vi "Step_Forward.vi"(3 "error in":errorcluster, 4 "Data in":T1, 5 "Step control reference in":refnum<vi>) -> (0 "error out":errorcluster, 1 "Data out":T1, 2 "Step control reference out":refnum<vi>)   [LabVIEW 2015]
uses:
  Type_Defs/Data.ctl
  Type_Defs/Diagnostics.ctl
  Type_Defs/Systems.ctl
  Step_Vis/Steps.lvlib
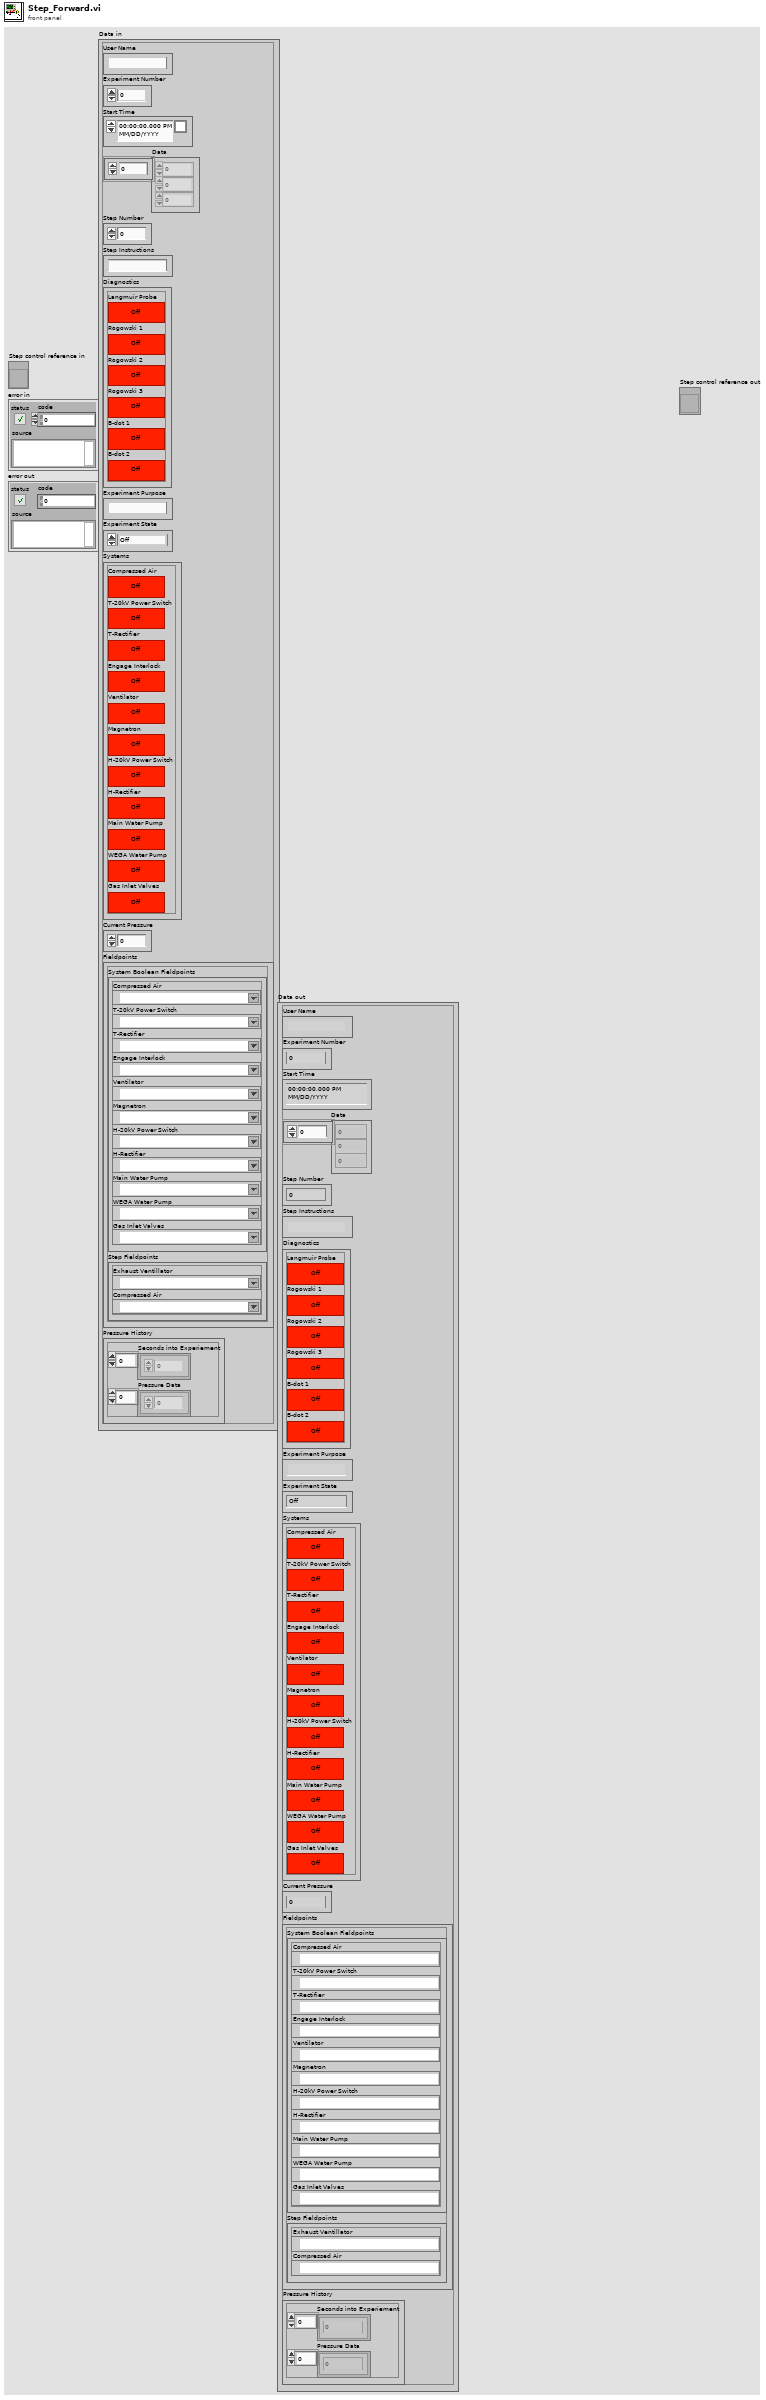
[diagram p1: front panel]
types:
  T1 = typedef "Data.ctl" = cluster{"User Name":string, "Experiment Number":i32, "Start Time":timestamp, "Data":dbl[], "Step Number":i32, "Step Instructions":string, "Diagnostics":T2, "Experiment Purpose":string, "Experiment State":enum16{"Off", "Setting Up", "Ready", "In Progress", "Shutting Down"}, "Systems":T3, "Current Pressure":dbl, "Fieldpoints":cluster{"System Boolean Fieldpoints":cluster{"Compressed Air":refnum<k21>, "T-20kV Power Switch":refnum<k21>, "T-Rectifier":refnum<k21>, "Engage Interlock":refnum<k21>, "Ventilator":refnum<k21>, "Magnetron":refnum<k21>, "H-20kV Power Switch":refnum<k21>, "H-Rectifier":refnum<k21>, "Main Water Pump":refnum<k21>, "WEGA Water Pump":refnum<k21>, "Gas Inlet Valves":refnum<k21>}, "Step Fieldpoints":cluster{"Exhaust Ventillator":refnum<k21>, "Compressed Air":refnum<k21>}}, "Pressure History":cluster{"Seconds into Experiement":i32[], "Pressure Data":dbl[]}}
  T2 = typedef "Diagnostics.ctl" = cluster{"Langmuir Probe":bool, "Rogowski 1":bool, "Rogowski 2":bool, "Rogowski 3":bool, "B-dot 1":bool, "B-dot 2":bool}
  T3 = typedef "Systems.ctl" = cluster{"Compressed Air":bool, "T-20kV Power Switch":bool, "T-Rectifier":bool, "Engage Interlock":bool, "Ventilator":bool, "Magnetron":bool, "H-20kV Power Switch":bool, "H-Rectifier":bool, "Main Water Pump":bool, "WEGA Water Pump":bool, "Gas Inlet Valves":bool}
  T4 = enum16{"Off", "Setting Up", "Ready", "In Progress", "Shutting Down"}
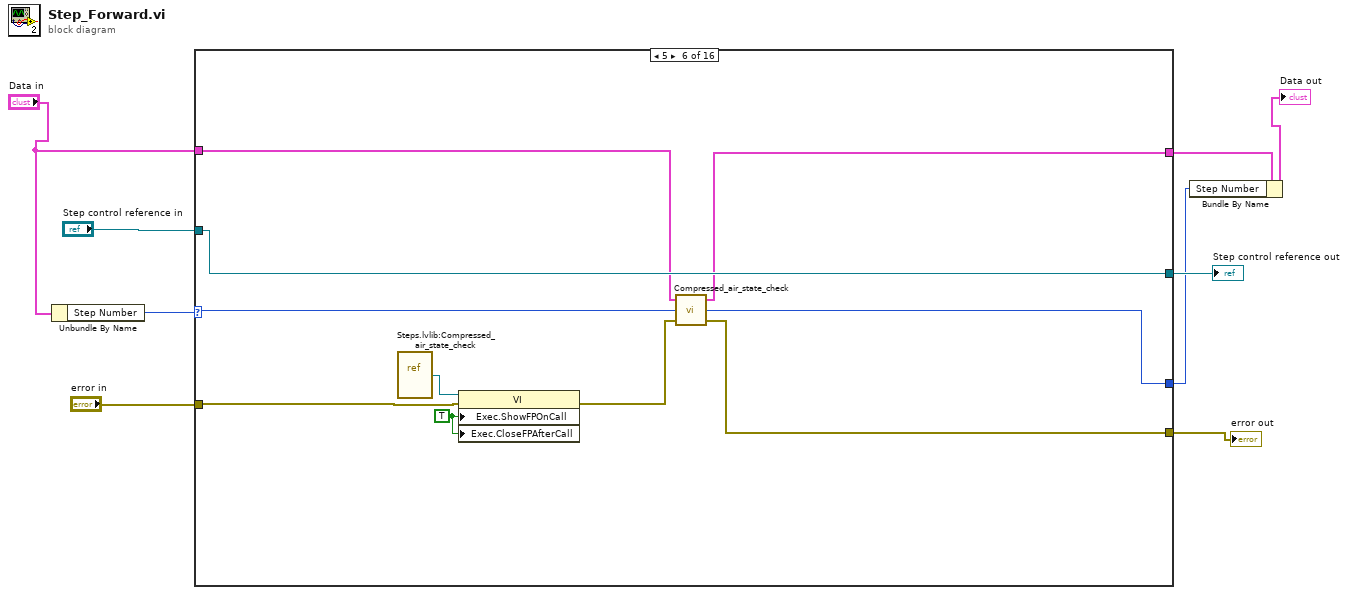
[diagram p0: block diagram]
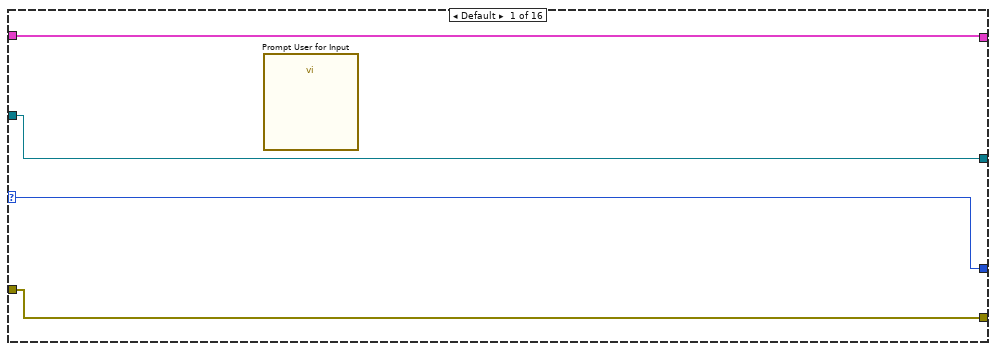
[diagram p2: hidden frame]
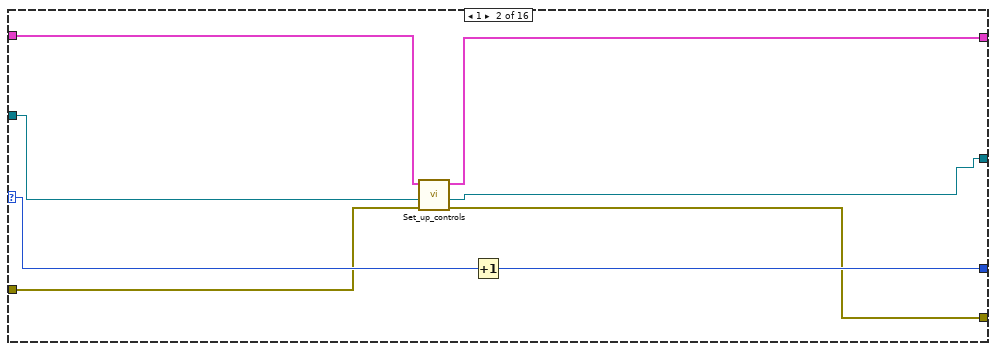
[diagram p3: hidden frame]
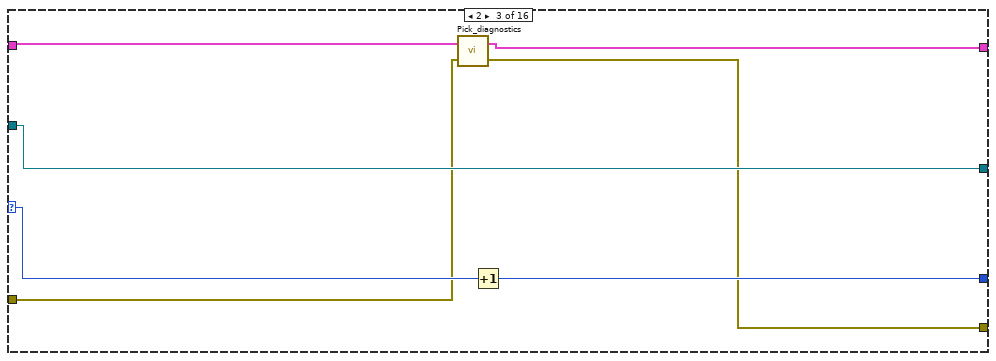
[diagram p4: hidden frame]
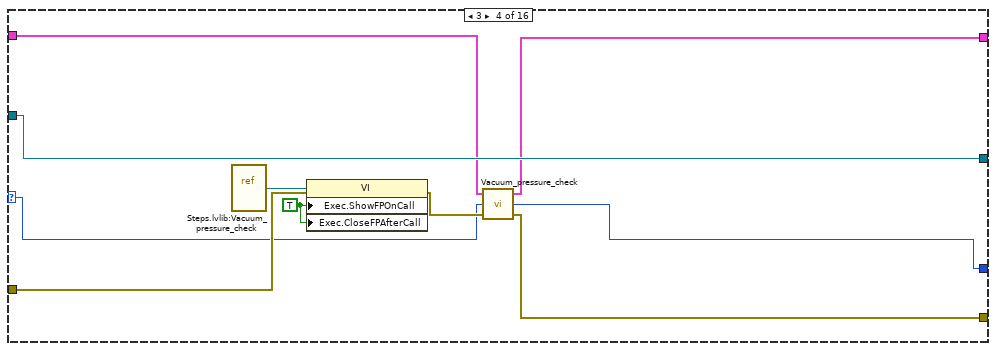
[diagram p5: hidden frame]
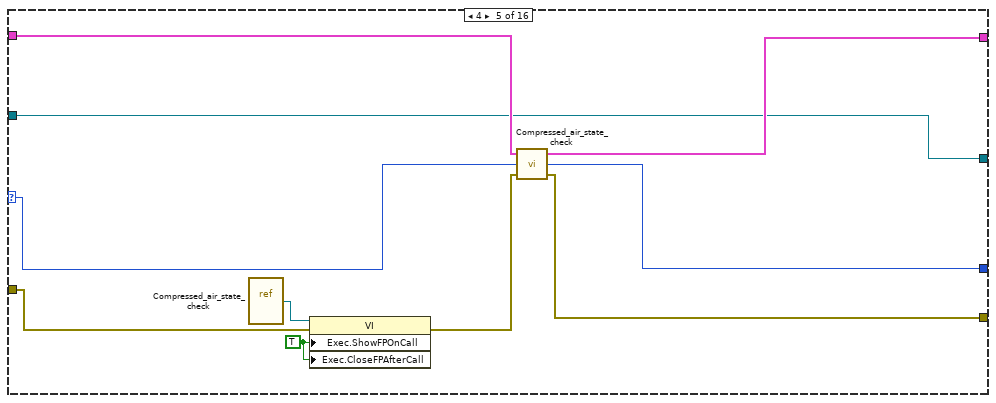
[diagram p6: hidden frame]
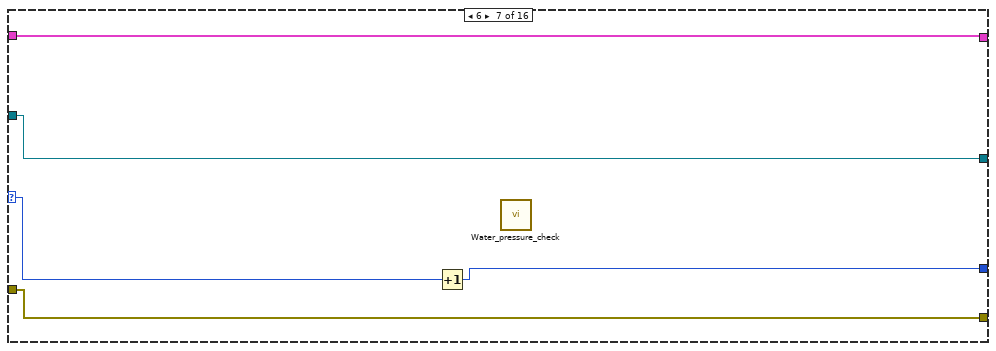
[diagram p7: hidden frame]
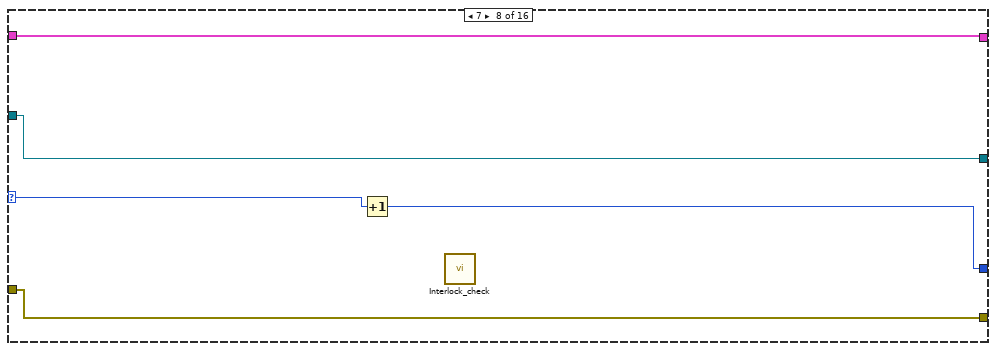
[diagram p8: hidden frame]
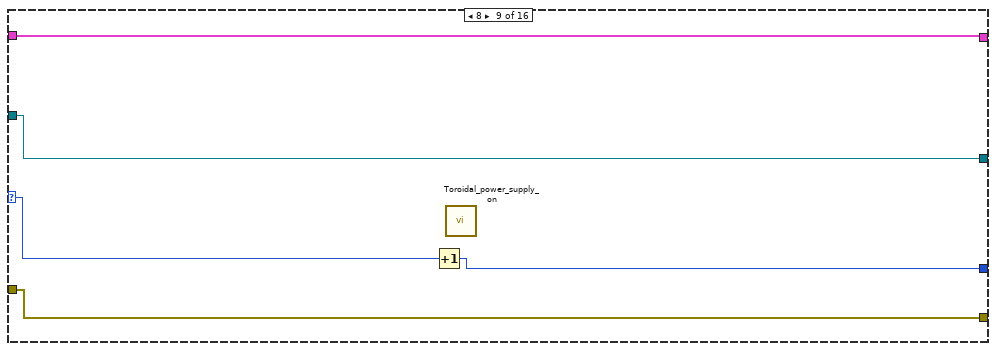
[diagram p9: hidden frame]
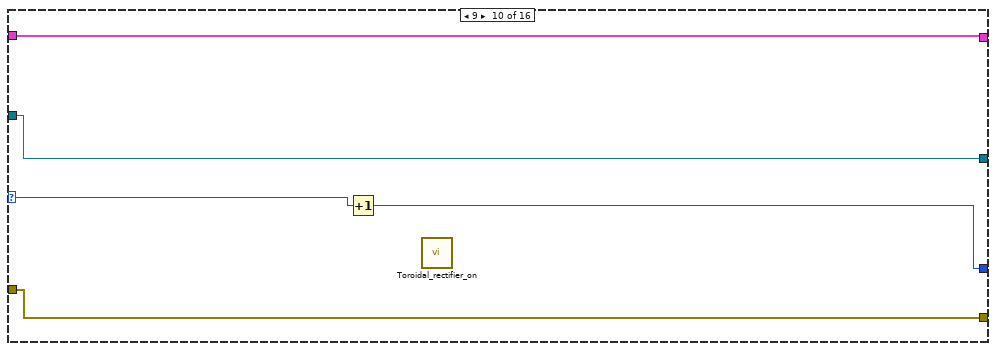
[diagram p10: hidden frame]
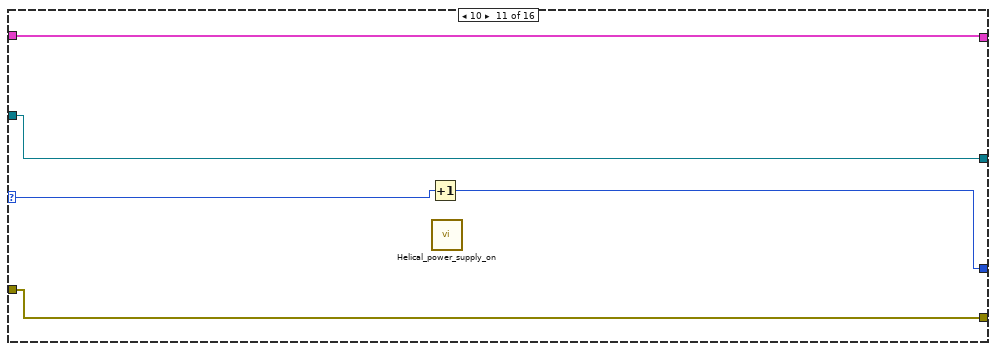
[diagram p11: hidden frame]
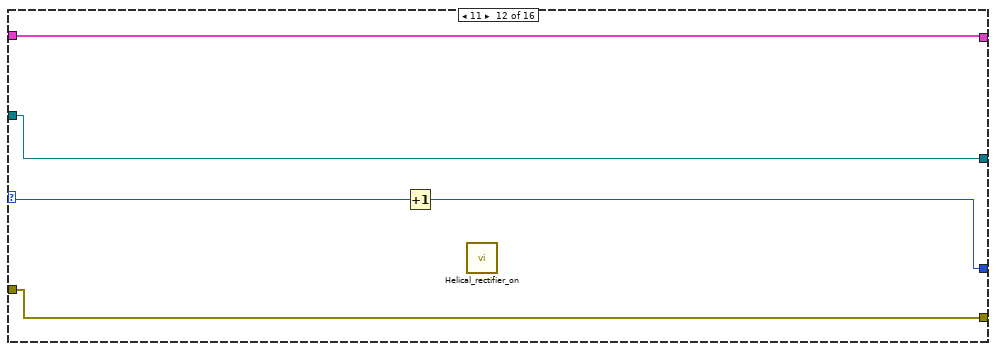
[diagram p12: hidden frame]
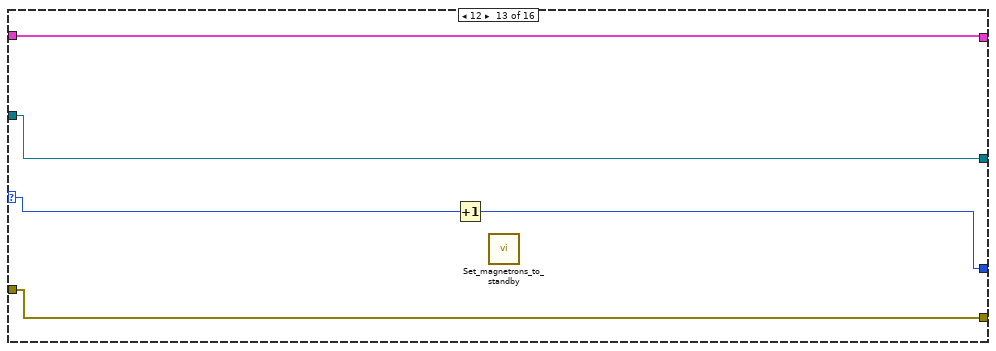
[diagram p13: hidden frame]
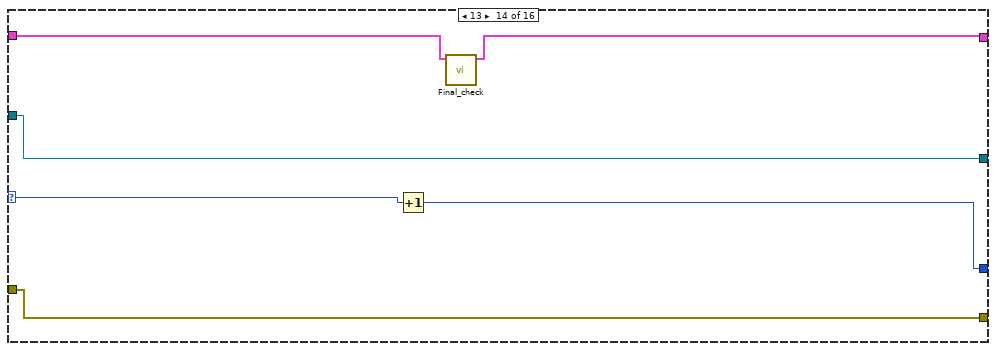
[diagram p14: hidden frame]
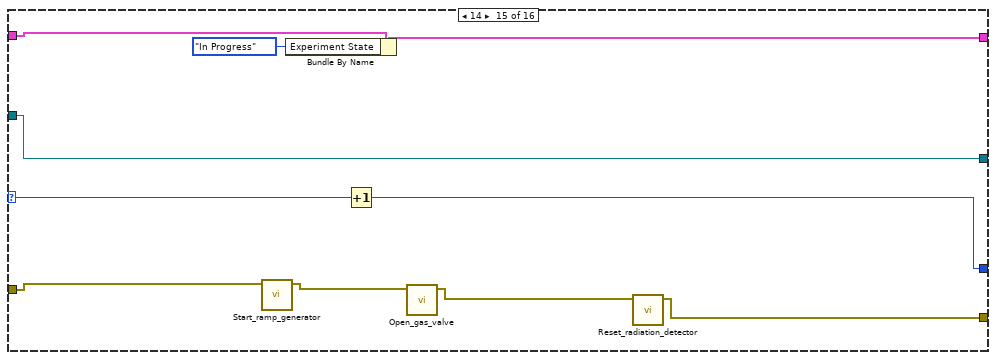
[diagram p15: hidden frame]
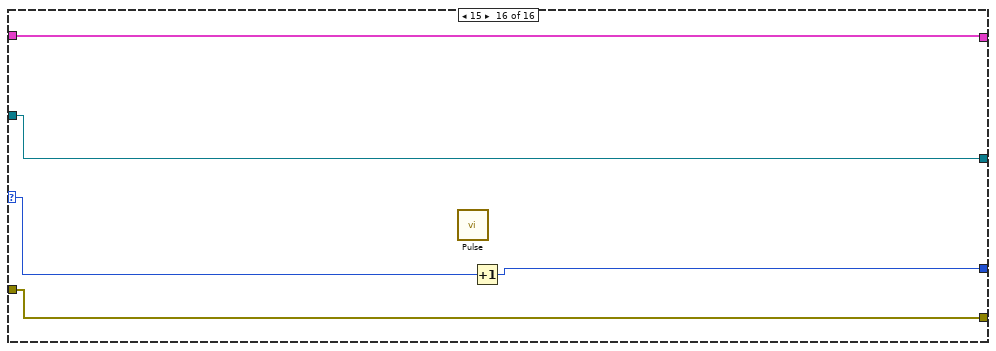
[diagram p16: hidden frame]
diagram:
  n1 = Unbundle By Name("Data in") -> ("Step Number"=w5:i32)
  n2 = case shown="5" w5 {
    selector: w5 -> [w12 w21 w28 w29 w45 w57 w59 w65 w69 w75 w80 w85 w89 w97 w107 w110]
    tunnel: "Step control reference in" -> [w13 w17 w26 w38 w44 w58 w63 w68 w73 w78 w83 w88 w93 w99 w109 w114]
    tunnel: [w13 w14 w26 w38 w44 w58 w63 w68 w73 w78 w83 w88 w93 w99 w109 w114] -> w8
    tunnel: [w12 w20 w27 w30 w46 w53 w60 w64 w70 w74 w79 w84 w90 w96 w108 w111] -> w3
    tunnel: "error in" -> [w11 w19 w25 w36 w41 w49 w62 w67 w72 w77 w82 w87 w92 w98 w106 w113]
    tunnel: [w11 w18 w24 w34 w43 w54 w62 w67 w72 w77 w82 w87 w92 w98 w103 w113] -> w6
    tunnel: "Data in" -> [w10 w16 w23 w32 w48 w55 w61 w66 w71 w76 w81 w86 w91 w95 w102 w112]
    tunnel: [w10 w15 w22 w31 w47 w56 w61 w66 w71 w76 w81 w86 w91 w94 w101 w112] -> w4
    frame Default {
      n3 = call "Prompt User for Input"() -> ()  [unwired: 18 in, 2 out]
    }
    frame 1 {
      n4 = call "Set_up_controls.vi"("error in"=w19, "reference"=w17, "Data in"=w16) -> ("error out"=w18:errorcluster, "reference out"=w14:refnum<vi>, "Data out"=w15:T1)  [unwired: 1 in, 1 out]
      n5 = Increment(x=w21) -> (x+1=w20:i32)
    }
    frame 2 {
      n6 = call "Pick_diagnostics.vi"("error in (no error)"=w25, "Data In"=w23) -> ("error out"=w24:errorcluster, "Data Out"=w22:T1)
      n7 = Increment(x=w28) -> (x+1=w27:i32)
    }
    frame 3 {
      w33 = TRUE ("Execution:Show Front Panel On Call")
      n8 = vi-ref "Steps.lvlib:Vacuum_pressure_check.vi"() -> (w37:refnum<vi>)
      n9 = property class="VI"(reference=w37, error in=w36, "Exec.ShowFPOnCall"=w33, "Exec.CloseFPAfterCall"=w33) -> (error out=w35:errorcluster)  [unwired: 1 out]
      n10 = call "Vacuum_pressure_check.vi"("error in"=w35, "Step Number in"=w29, "Data in"=w32) -> ("error out"=w34:errorcluster, "Step Number out"=w30:i32, "Data out"=w31:T1)
    }
    frame 4 {
      w42 = TRUE ("Execution:Show Front Panel On Call")
      n11 = vi-ref "Compressed_air_state_check.vi"() -> (w39:refnum<vi>)
      n12 = property class="VI"(reference=w39, error in=w41, "Exec.ShowFPOnCall"=w42, "Exec.CloseFPAfterCall"=w42) -> (error out=w40:errorcluster)  [unwired: 1 out]
      n13 = call "Compressed_air_state_check.vi"("error in"=w40, "Step Number in"=w45, "Data in"=w48) -> ("error out"=w43:errorcluster, "Step Number out"=w46:i32, "Data out"=w47:T1)
    }
    frame 5 {
      w52 = TRUE ("Execution:Show Front Panel On Call")
      n14 = vi-ref "Steps.lvlib:Compressed_air_state_check.vi"() -> (w51:refnum<vi>)
      n15 = property class="VI"(reference=w51, error in=w49, "Exec.ShowFPOnCall"=w52, "Exec.CloseFPAfterCall"=w52) -> (error out=w50:errorcluster)  [unwired: 1 out]
      n16 = call "Compressed_air_state_check.vi"("error in"=w50, "Step Number in"=w57, "Data in"=w55) -> ("error out"=w54:errorcluster, "Step Number out"=w53:i32, "Data out"=w56:T1)
    }
    frame 6 {
      n17 = Increment(x=w59) -> (x+1=w60:i32)
      n18 = call "Water_pressure_check.vi"() -> ()  [unwired: 12 in]
    }
    frame 7 {
      n19 = Increment(x=w65) -> (x+1=w64:i32)
      n20 = call "Interlock_check.vi"() -> ()  [unwired: 12 in]
    }
    frame 8 {
      n21 = Increment(x=w69) -> (x+1=w70:i32)
      n22 = call "Toroidal_power_supply_on.vi"() -> ()  [unwired: 12 in]
    }
    frame 9 {
      n23 = Increment(x=w75) -> (x+1=w74:i32)
      n24 = call "Toroidal_rectifier_on.vi"() -> ()  [unwired: 12 in]
    }
    frame 10 {
      n25 = Increment(x=w80) -> (x+1=w79:i32)
      n26 = call "Helical_power_supply_on.vi"() -> ()  [unwired: 12 in]
    }
    frame 11 {
      n27 = Increment(x=w85) -> (x+1=w84:i32)
      n28 = call "Helical_rectifier_on.vi"() -> ()  [unwired: 12 in]
    }
    frame 12 {
      n29 = Increment(x=w89) -> (x+1=w90:i32)
      n30 = call "Set_magnetrons_to_standby.vi"() -> ()  [unwired: 12 in]
    }
    frame 13 {
      n31 = Increment(x=w97) -> (x+1=w96:i32)
      n32 = call "Final_check.vi"("Data in"=w95) -> ("Data out"=w94:T1)  [unwired: 10 in]
    }
    frame 14 {
      n33 = call "Start_ramp_generator.vi"("error in"=w106) -> ("error out"=w105:errorcluster)  [unwired: 10 in]
      n34 = Bundle By Name(cluster=w102, "Experiment State"=T4."In Progress") -> (w101:T1)
      n35 = Increment(x=w107) -> (x+1=w108:i32)
      n36 = call "Open_gas_valve.vi"("error in"=w105) -> ("error out"=w104:errorcluster)  [unwired: 10 in]
      n37 = call "Reset_radiation_detector.vi"("error in"=w104) -> ("error out"=w103:errorcluster)  [unwired: 10 in]
    }
    frame 15 {
      n38 = call "Pulse.vi"() -> ()  [unwired: 12 in]
      n39 = Increment(x=w110) -> (x+1=w111:i32)
    }
  }
  "Step control reference out" <- w8
  "error out" <- w6
  n40 = Bundle By Name(cluster=w4, "Step Number"=w3) -> (→"Data out":T1)
